vi "Sort 2D Cell details Array.vi"(9 "Column descending? array":bool[](array[boolean]), 10 "Column priority array":dbl[](array[numeric]), 11 "Unsorted Array":string[][](array[string])) -> (3 "Sorted Array":string[][](array[string]))   [LabVIEW 2011]
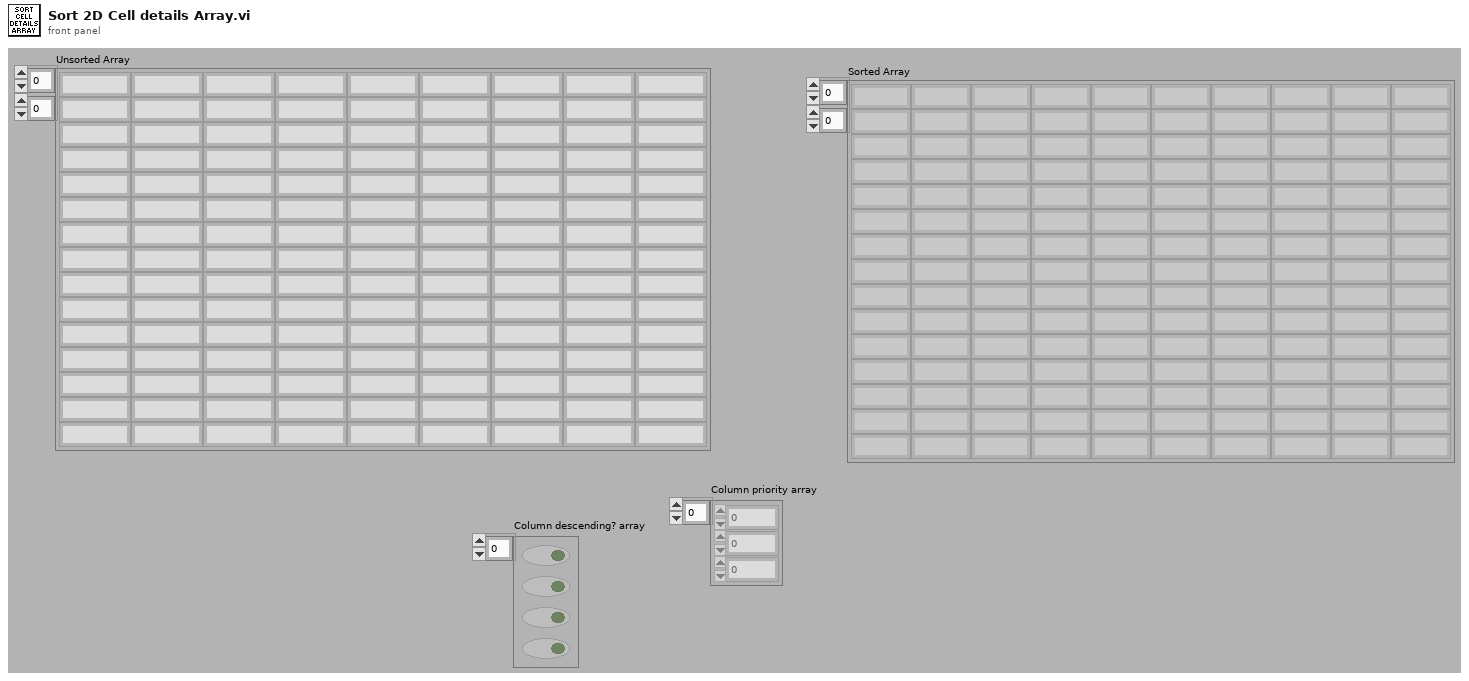
[diagram p1: front panel]
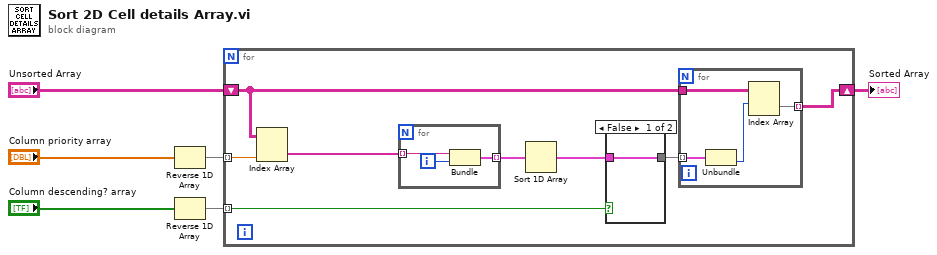
[diagram p0: block diagram]
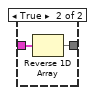
[diagram p2: hidden frame]
diagram:
  n1 = Reverse 1D Array(array="Column priority array") -> (reversed array=w6:dbl[])
  n2 = Reverse 1D Array(array="Column descending? array") -> (reversed array=w5:bool[])
  n3 = for {
    shift-right: [w11] -> w2
    shift-left: "Unsorted Array" -> [w13]
    tunnel: w6 -> [w12] mode=indexing
    tunnel: w5 -> [w7] mode=indexing
    n4 = Index Array(array=w13, index (col)=w12) -> (element=w10:string[])  [unwired: 1 in]
    n5 = for {
      tunnel: w10 -> [w23] mode=indexing
      tunnel: [w24] -> w14 mode=indexing
      i -> [w22]
      n6 = Bundle("String"=w23, w22) -> (w24:cluster{"String":string, i32})  [unwired: 1 out]
    }
    n7 = Sort 1D Array(array=w14) -> (sorted array=w9:cluster{"String":string, i32}[])
    n8 = case shown="False" w7 {
      tunnel: w9 -> [w15 w17]
      tunnel: [w15 w16] -> w8
      frame False {
      }
      frame True {
        n9 = Reverse 1D Array(array=w17) -> (reversed array=w16:cluster{"String":string, i32}[])
      }
    }
    n10 = for {
      tunnel: w8 -> [w21] mode=indexing
      tunnel: w13 -> [w20]
      tunnel: [w18] -> w11 mode=indexing
      n11 = Unbundle(w21) -> (w19:i32)  [unwired: 1 out]
      n12 = Index Array(array=w20, index (row)=w19) -> (element=w18:string[])  [unwired: 1 in]
    }
  }
  "Sorted Array" <- w2
